vi "Set Trigger.vi"(8 "error in (no error)":errorcluster, 11 "CCDCamera in":refnum<class "CCDCamera.lvclass">) -> (0 "error out":errorcluster, 3 "CCDCamera out":refnum<class "CCDCamera.lvclass">)   [LabVIEW 2018, in "CCDCamera.lvclass"]
uses:
  CCDCamera.lvclass
  C:/Users/observer/Desktop/SPARC4_ACS/Simulated_CCD_Camera/Simulated_CCD_Camera.lvclass
  Simulated_CCD_Camera/Simulated_CCD_Camera.lvclass/Simulated_CCD_Camera.ctl
  Simulated_CCD_Camera/Simulated_CCD_Camera.lvclass
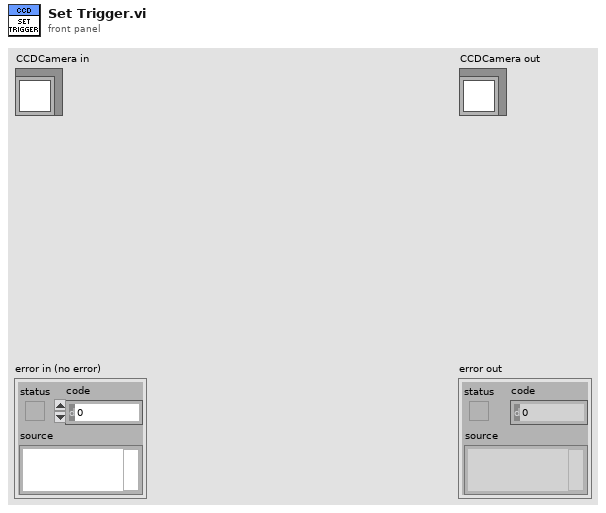
[diagram p1: front panel]
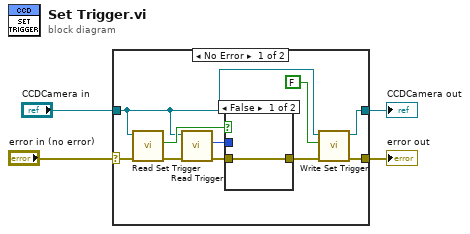
[diagram p0: block diagram]
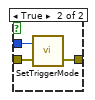
[diagram p2: hidden frame]
diagram:
  n1 = case shown="No Error" "error in (no error)" {
    selector: "error in (no error)" -> [w12 w20]
    tunnel: [w7 w20] -> w3
    tunnel: [w5 w19] -> w1
    tunnel: "CCDCamera in" -> [w6 w19]
    frame No Error {
      n2 = call "Read Set Trigger.vi"("error in (no error)"=w12, "Simulated_CCD_Camera in"=w6) -> ("error out"=w11:errorcluster, "Set Trigger"=w13:bool)  [unwired: 7 in, 1 out]
      n3 = call "Read Trigger.vi"("error in (no error)"=w11, "CCDCamera in"=w6) -> ("error out"=w10:errorcluster, "Trigger"=w14:u16)  [unwired: 7 in, 1 out]
      n4 = case shown="False" w13 {
        tunnel: [w15 w18] -> w8
        tunnel: w10 -> [w15 w17]
        tunnel: w14 -> [_ w16]
        frame False {
        }
        frame True {
          n5 = call <userlib>:"SetTriggerMode.vi"("error in (no error)"=w17, "mode"=w16) -> ("error out"=w18:errorcluster)  [unwired: 1 out]
        }
      }
      n6 = call "Write Set Trigger.vi"("error in (no error)"=w8, "Set Trigger"=FALSE ("CCD Config.Set Trigger"), "Simulated_CCD_Camera in"=w6) -> ("error out"=w7:errorcluster, "Simulated_CCD_Camera out"=w5:refnum<class "CCDCamera.lvclass">)  [unwired: 7 in]
    }
    frame Error {
    }
  }
  "error out" <- w3
  "CCDCamera out" <- w1
